vi "licdf version.vi"(8 "error in (no error)":errorcluster, 9 "out_patch":i32, 10 "out_minor":i32, 11 "out_major":i32) -> (0 "error out":errorcluster, 1 "out_patch out":i32, 2 "out_minor out":i32, 3 "out_major out":i32, 5 "function return":i32)   [LabVIEW 2026, in "keynub_licdongle.lvlib"]
doc: "int32_t licdf_version(int32_t *out_major, int32_t *out_minor, int32_t *out_patch);"
uses:
  keynub_licdongle.lvlib
  natives/win-x64/keynub_licdongle_flat.dll
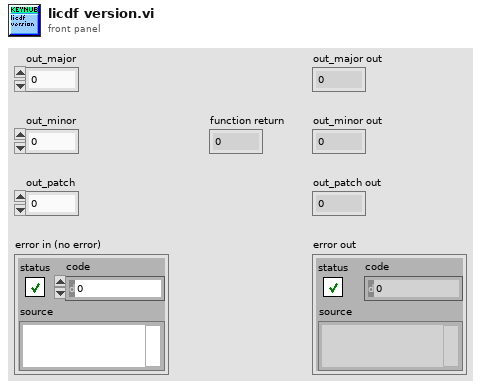
[diagram p1: front panel]
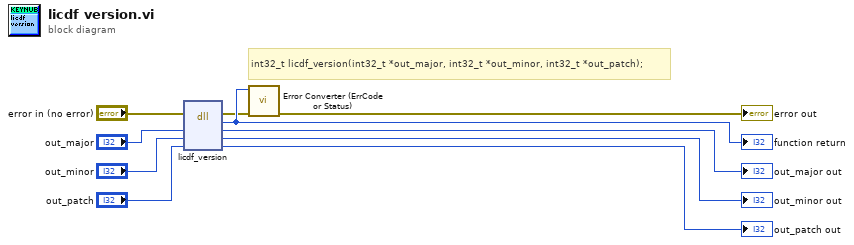
[diagram p0: block diagram]
diagram:
  # "int32_t licdf_version(int32_t *out_major, int32_t *out_minor, int32_t *out_patch);"
  n1 = dll-call lib="C:/Austausch/KeyNub/LicenseDongle-PublicSDK/natives/win-x64/keynub_licdongle_flat.*" fn="licdf_version"(error in="error in (no error)", "out_major"="out_major", "out_minor"="out_minor", "out_patch"="out_patch") -> (error out=w2:errorcluster, w10:i32, "out_major"=→"out_major out":i32, "out_minor"=→"out_minor out":i32, "out_patch"=→"out_patch out":i32)  [unwired: 2 in, 1 out]
  "function return" <- w10
  n2 = call "Error Converter (ErrCode or Status).vi"("error in (no error)"=w2, "error code"=w10) -> ("error out"=→"error out":errorcluster)  [unwired: 9 in]
